vi "save_datapoint.vi"(0 "current value":dbl, 1 "Sample number":i32, 2 "current time of measurement":timestamp, 3 "Sensor type":T1) -> ()   [LabVIEW 2012]
uses:
  SensorTypes.ctl
  globalVariables.vi
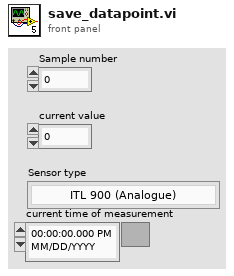
[diagram p1: front panel]
types:
  T1 = typedef "SensorTypes.ctl" = enum16{"ITL 900 (Analogue)", "CAB 300-C SP3 (CAN)", "xyz TODO (PWM)", "xyz TODO (LIN)", "xyz TODO (Analogue)"}
  T2 = typedef "TimeValue.ctl" = cluster{"Time of measurement":timestamp, "Current value":dbl}
  T3 = typedef "Semaphore RefNum" = refnum<k1>
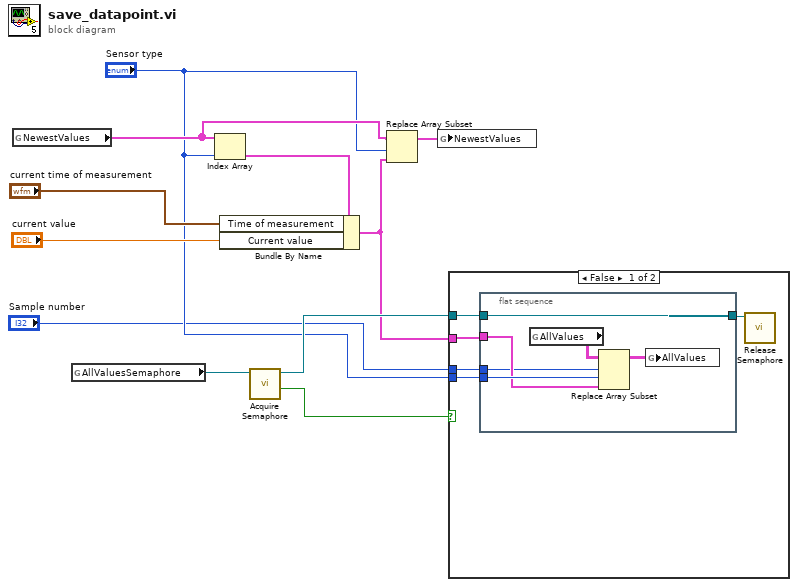
[diagram p0: block diagram]
diagram:
  n1 = global read "globalVariables.vi" "NewestValues"() -> (w9:T2[])
  n2 = global read "globalVariables.vi" "AllValuesSemaphore"() -> (w6:T3)
  n3 = Index Array(array=w9, index="Sensor type") -> (element=w8:T2)
  n4 = Bundle By Name(cluster=w8, "Time of measurement"="current time of measurement", "Current value"="current value") -> (w2:T2)
  n5 = call <vilib>:"Acquire Semaphore.vi"("semaphore"=w6) -> ("timed out"=w4:bool, "semaphore out"=w5:T3)  [unwired: 4 in, 1 out]
  n6 = Replace Array Subset(array=w9, new element=w2, index="Sensor type") -> (w10:T2[])
  n7 = global write "globalVariables.vi" "NewestValues"(w10) -> ()
  n8 = case shown="False" w4 {
    tunnel: w5 -> [w16 _]
    tunnel: "Sample number" -> [w14 _]
    tunnel: "Sensor type" -> [w13 _]
    tunnel: w2 -> [w12 _]
    frame False {
      n9 = flat-sequence {
        tunnel: w16 -> [w22]
        tunnel: [w22] -> w15
        tunnel: w14 -> [w17]
        tunnel: w13 -> [w19]
        tunnel: w12 -> [w18]
        frame #0 {
          n10 = global read "globalVariables.vi" "AllValues"() -> (w21:T2[][])
          n11 = Replace Array Subset(array=w21, new element=w18, index (row)=w17, index (col)=w19) -> (w20:T2[][])
          n12 = global write "globalVariables.vi" "AllValues"(w20) -> ()
        }
      }
      n13 = call <vilib>:"Release Semaphore.vi"("semaphore"=w15) -> ()  [unwired: 5 in, 2 out]
    }
    frame True {
    }
  }
